vi "TagDB For Control Reference.vi"() -> ()   [LabVIEW 2017]
uses:
  db75e40e-e2ce-4478-aeb2-ba442eae1a36.vi
  6e72737a-719b-451f-8a50-03ef03344deb.vi
  4295ea48-1fc4-4cd1-998c-9dd8fac1b23c.vi
  85ab2e25-d076-4b48-b8d4-5749372e6319.vi
  a6b6e2a6-547b-4695-ab8c-6de39fa5d339.vi
  6af427bf-a3b3-4747-adc4-f86c2d92cb3a.vi
  818069fb-06b6-4ca3-92f6-007415f4d322.vi
  TagDB/_Support/DataAccess/data-Write.vi
  TagDB/_Support/Error/_[error50000]Invalid DB REF.vi
  TagDB/_Support/DataAccess/TagDB Ref to DVR.vi
  TagDB/_Support/DataAccess/_NameCacher.vi
  TagDB/_Support/Error/_[error50002]Invalid DataType.vi
  TagDB/_Support/URL/TRIM-BOTH-SPACE.vi
  TagDB/_Support/Change Detector/TagDB dbChanged.vi
  TagDB/_Support/Error/_Clear Errors.vi
  6af427bf-a3b3-4747-adc4-f86c2d92cb3a.vi/29b2ea6d-6d7f-4e4a-ad31-a5cb760462c7.vi
  TagDB/API/TagDB-Status.vi
  818069fb-06b6-4ca3-92f6-007415f4d322.vi/29b2ea6d-6d7f-4e4a-ad31-a5cb760462c7.vi
  TagDB/_Support/DataAccess/_datatypeChecker.vi
  TagDB/_Support/Change Detector/TagDB ChangeFlag.vi
  <vilib>/Utility/Data Type/Get Type Information.vi
  TagDB/_Support/Error/_Build Error Cluster.vi
  TagDB/TagDB.lvlib
panel:
  out "Array 2":dbl[](array[numeric])=[123.0]
  out "Array":string[](array[string])=["Numeric0", "Numeric1"]
  in  "Numeric1":string="abc"
  out "Value 0":dbl=123.0
  out "Class Name":string="Digital"
  in  "Numeric0":dbl=123.0
  out "label":string="Numeric0"
  # "1"
  # "2"
  # "3"
  # "4"
  # "5"
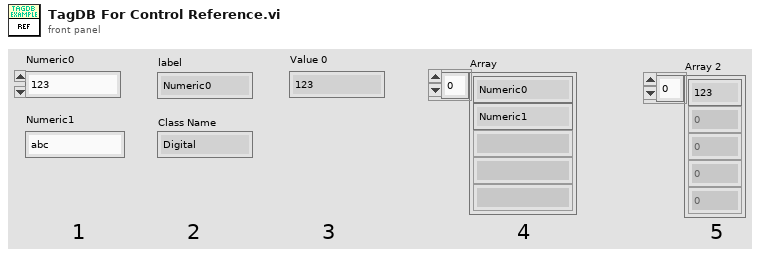
[diagram p1: front panel]
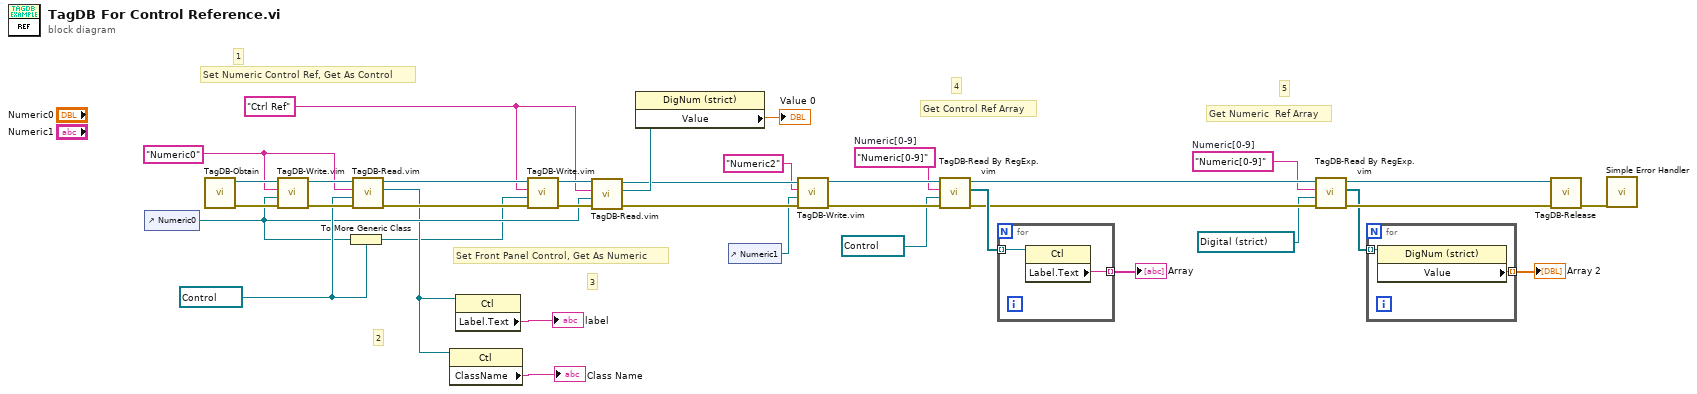
[diagram p0: block diagram]
diagram:
  w2 = "Numeric[0-9]"  # Numeric[0-9]
  w3 = "Numeric[0-9]"  # Numeric[0-9]
  w27 = "Ctrl Ref"
  w25 = refnum<vi> refnum ("value")
  w34 = "Numeric0"
  # "5"
  # "4"
  # "1"
  # "3"
  # "2"
  # "Get Numeric  Ref Array"
  # "Get Control Ref Array"
  # "Set Front Panel Control, Get As Numeric"
  # "Set Numeric Control Ref, Get As Control"
  n1 = control-ref of="Numeric0"() -> (w23:refnum<vi>)
  n2 = call "TagDB-Obtain.vi"() -> ("error out"=w35:errorcluster, "TagDB"=w36:refnum<k1>)  [unwired: 5 in, 1 out]
  n3 = call "TagDB-Write.vim"("error in (no error)"=w35, "Value"=w23, "tag"=w34, "TagDB"=w36) -> ("error out"=w33:errorcluster, "TagDB(dup)"=w37:refnum<k1>)  [unwired: 5 in, 1 out]
  n4 = To More Generic Class(target class=w25, reference=w23) -> (generic class reference=w1:refnum<vi>)
  n5 = call "TagDB-Read.vim"("error in (no error)"=w33, "Type(empty to read as variant)"=w25, "name"=w34, "TagDB"=w37) -> ("error out"=w28:errorcluster, "Value"=w21:refnum<vi>, "TagDB(dup)"=w29:refnum<k1>)  [unwired: 2 in, 3 out]
  n6 = property class="Ctl"(reference=w21) -> ("ClassName"=→"Class Name":string)  [unwired: 1 in, 2 out]
  n7 = property class="Ctl"(reference=w21) -> ("Label.Text"=→"label":string)  [unwired: 1 in, 2 out]
  n8 = call "TagDB-Write.vim"("error in (no error)"=w28, "Value"=w1, "tag"=w27, "TagDB"=w29) -> ("error out"=w31:errorcluster, "TagDB(dup)"=w30:refnum<k1>)  [unwired: 5 in, 1 out]
  n9 = call "TagDB-Read.vim"("error in (no error)"=w31, "Type(empty to read as variant)"=w23, "name"=w27, "TagDB"=w30) -> ("error out"=w19:errorcluster, "Value"=w24:refnum<vi>, "TagDB(dup)"=w20:refnum<k1>)  [unwired: 2 in, 3 out]
  n10 = property class="DigNum (strict)"(reference=w24) -> ("Value"=→"Value 0":dbl)  [unwired: 1 in, 2 out]
  n11 = control-ref of="Numeric1"() -> (w18:refnum<vi>)
  n12 = call "TagDB-Write.vim"("error in (no error)"=w19, "Value"=w18, "tag"="Numeric2", "TagDB"=w20) -> ("error out"=w15:errorcluster, "TagDB(dup)"=w16:refnum<k1>)  [unwired: 5 in, 1 out]
  n13 = call "TagDB-Read By RegExp.vim"("error in (no error)"=w15, "Type"=refnum<vi> refnum ("value"), "RegExp"=w3, "DB Ref"=w16) -> ("error out"=w8:errorcluster, "value"=w13:refnum<vi>[], "DB Ref(dup)"=w9:refnum<k1>)  [unwired: 4 in, 1 out]
  n14 = for {
    tunnel: w13 -> [w39] mode=indexing
    tunnel: [w38] -> w12 mode=indexing
    n15 = property class="Ctl"(reference=w39) -> ("Label.Text"=w38:string)  [unwired: 1 in, 2 out]
  }
  "Array" <- w12
  n16 = call "TagDB-Read By RegExp.vim"("error in (no error)"=w8, "Type"=refnum<vi> refnum ("Numeric1"), "RegExp"=w2, "DB Ref"=w9) -> ("error out"=w11:errorcluster, "value"=w7:refnum<vi>[], "DB Ref(dup)"=w10:refnum<k1>)  [unwired: 4 in, 1 out]
  n17 = for {
    tunnel: w7 -> [w41] mode=indexing
    tunnel: [w40] -> w6 mode=indexing
    n18 = property class="DigNum (strict)"(reference=w41) -> ("Value"=w40:dbl)  [unwired: 1 in, 2 out]
  }
  "Array 2" <- w6
  n19 = call "TagDB-Release.vi"("error in (no error)"=w11, "TagDB"=w10) -> ("error out"=w4:errorcluster)  [unwired: 9 in]
  n20 = call <vilib>:"Simple Error Handler.vi"("error in (no error)"=w4) -> ()  [unwired: 4 in, 5 out]
